vi "Check LC&RF Size Equality.vi"(8 "Error In":errorcluster, 9 "Variables":string[](array[string]), 11 "Linked Channels in":cluster{"Variable Name":string, "GUID":string}[](array[cluster])) -> (0 "Error Out":errorcluster, 1 "Variables out":string[](array[string]), 3 "Linked Channels out":cluster{"Variable Name":string, "GUID":string}[](array[cluster]))   [LabVIEW 2018, in "Instrument Addon Scripting API.lvlib"]
uses:
  Instrument Addon Scripting API.lvlib
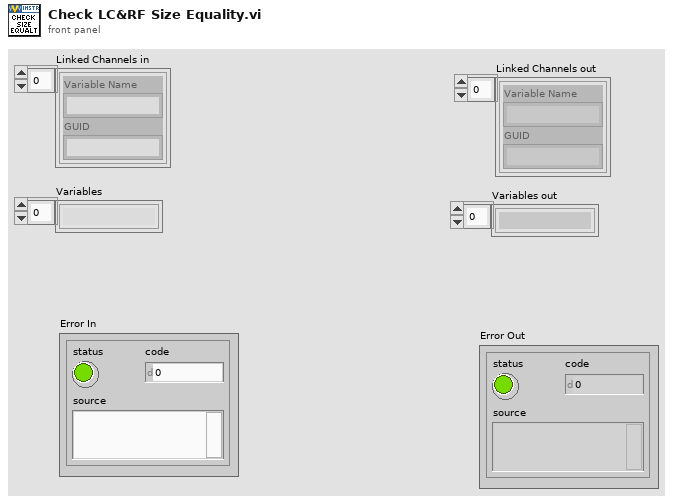
[diagram p1: front panel]
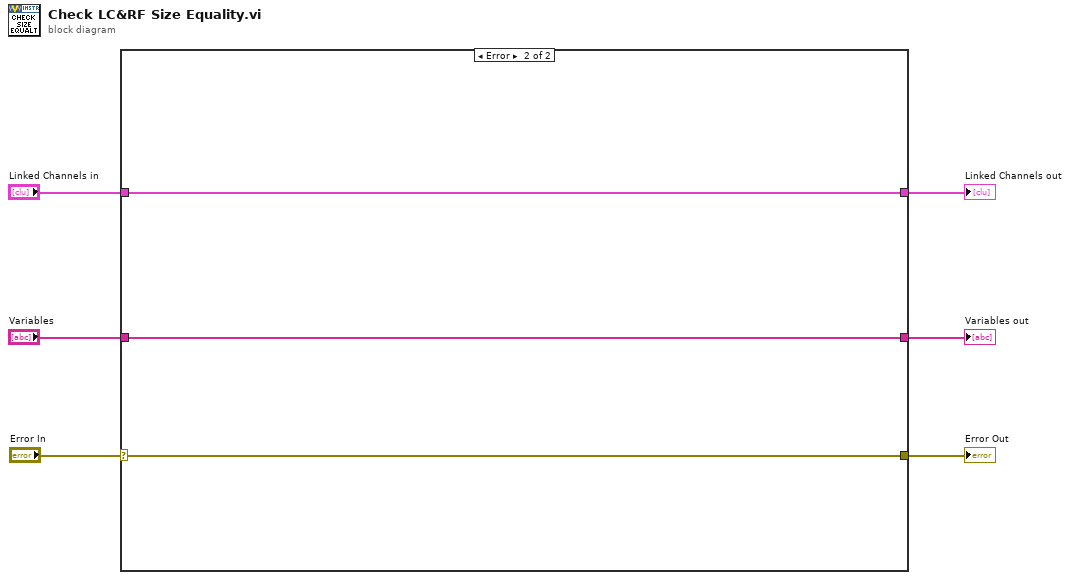
[diagram p0: block diagram]
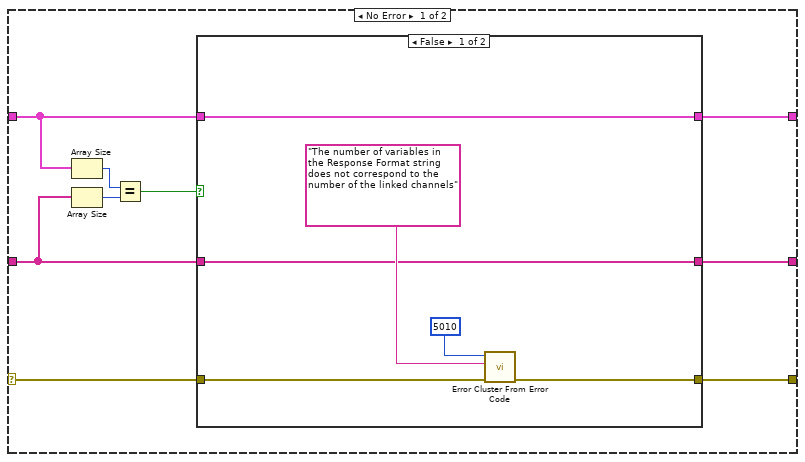
[diagram p2: hidden frame]
diagram:
  n1 = case shown="Error" "Error In" {
    selector: "Error In" -> [w12 w27]
    tunnel: "Variables" -> [w10 w25]
    tunnel: "Linked Channels in" -> [w9 w26]
    tunnel: [w11 w27] -> w3
    tunnel: [w8 w26] -> w2
    tunnel: [w7 w25] -> w1
    frame No Error {
      n2 = Array Size(array=w9) -> (size(s)=w15:i32)
      n3 = Array Size(array=w10) -> (size(s)=w14:i32)
      n4 = Equal?(x=w15, y=w14) -> (x = y?=w13:bool)
      n5 = case shown="False" w13 {
        tunnel: w12 -> [w19 w24]
        tunnel: [w18 w24] -> w11
        tunnel: w10 -> [w16 w22]
        tunnel: w9 -> [w17 w23]
        tunnel: [w17 w23] -> w8
        tunnel: [w16 w22] -> w7
        frame False {
          n6 = call <vilib>:"Error Cluster From Error Code.vi"("error in (no error)"=w19, "error message (\"\")"="The number of variables in the Response Format string does not correspond to the number of the linked channels" ("error message (\"\")"), "error code (0)"=5010) -> ("error out"=w18:errorcluster)  [unwired: 6 in]
        }
        frame True {
        }
      }
    }
    frame Error {
    }
  }
  "Error Out" <- w3
  "Linked Channels out" <- w2
  "Variables out" <- w1
